vi "Robot Main.vi"() -> ()   [LabVIEW 2014]
doc: "This VI implements the framework and scheduler for your robotics program. It should not be necessary to modify the framework. You are expected to add your code to the VIs called from Robot Main - the ones located in the Team Code folder within the project."
uses:
  <vilib>/Rock Robotics/WPI/Camera/WPI_CameraImageSize.ctl
  TypeDefs/SRE Enum.ctl
  <vilib>/Rock Robotics/WPI/DriverStation/WPI_DriverStationDerivedRobotMode.ctl
  Support Code/Robot Global Data.vi
  <vilib>/Rock Robotics/Network Tables/SD Read Boolean.vi
panel:
  in  "Limit":dbl=0.45
  in  "Image Size":T1=enum."320x240"
  in  "Enable Vision":bool
  in  "Finish":bool
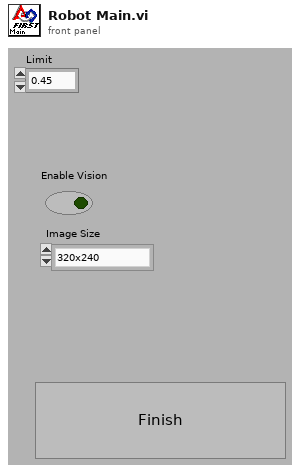
[diagram p1: front panel]
types:
  T1 = typedef "WPI_CameraImageSize.ctl" = enum16{"640x480", "320x240", "160x120", "Custom"}
  T2 = typedef "WPI_DriverStationDerivedRobotMode.ctl" = enum16{"Init", "Execute", "Stop"}
  T3 = typedef "SRE Enum.ctl" = enum16{"Start", "Run", "End"}
  T4 = cluster{"Speed":dbl, "Direction":dbl, "Rotation":dbl}
  T5 = enum16{"High", "Middle", "Low", "Really Low", "Stopped"}
  T6 = typedef "WPI_DriverStationMatch Info.ctl" = cluster{"Autonomous Elapsed Seconds":dbl, "TeleOp Elapsed Seconds":dbl, "Disabled Elapsed Seconds":dbl, "Visited Autonomous":bool, "Visited TeleOp":bool, "Visited Disabled":bool, "Autonomous Settings":cluster{"Autonomous Style":enum16{"Iterative", "Independent"}, "VI Refnum":refnum<vi>}}
  T7 = typedef "WPI_DriverStationRobotMode2.ctl" = enum16{"Autonomous Disabled", "Autonomous Enabled", "Teleop Disabled", "Teleop Enabled", "Disconnected", "Finish", "Test Disabled", "Test Enabled", "Emergency Stopped"}
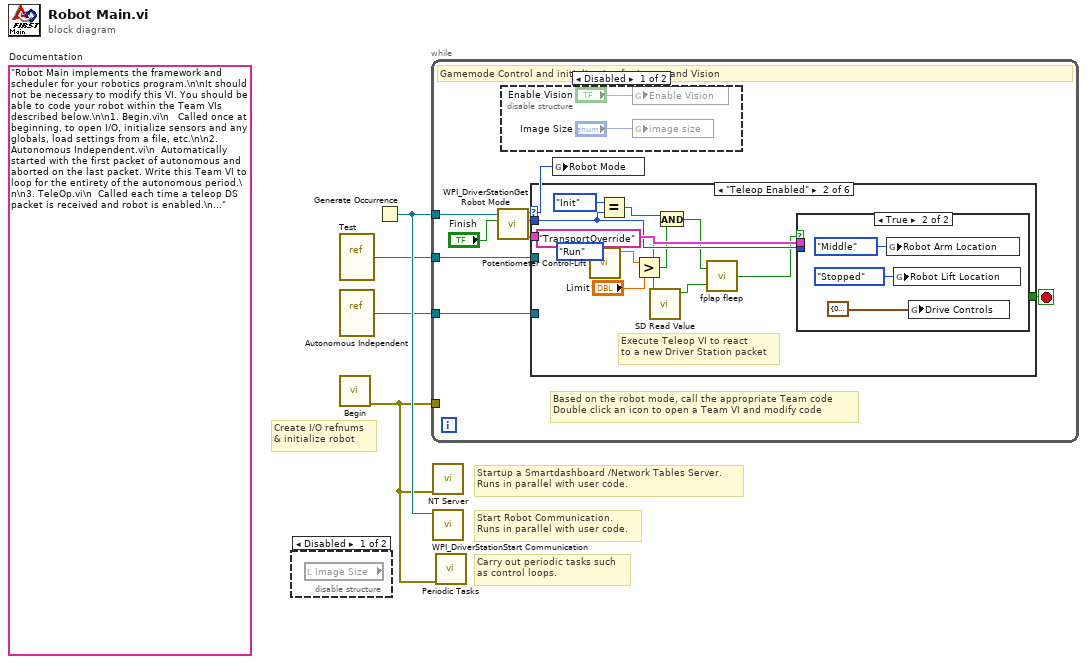
[diagram p0: block diagram]
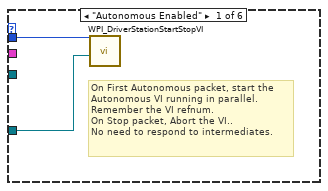
[diagram p4: hidden frame]
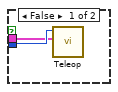
[diagram p5: hidden frame]
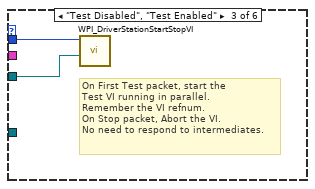
[diagram p6: hidden frame]
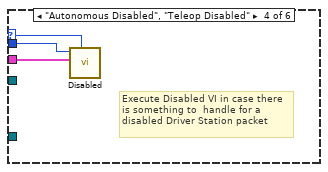
[diagram p7: hidden frame]
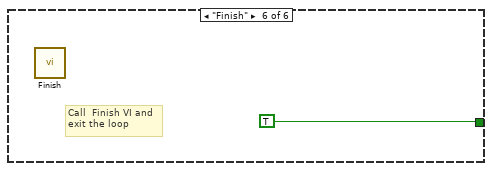
[diagram p9: hidden frame]
diagram:
  (unwired) "Robot Main implements the framework and scheduler for your robotics program.\n\nIt should not be necessary to modify this VI. You should be able to code your robot within the Team VIs described below.\n\n1. Begin.vi\n   Called once at beginning, to open I/O, initialize sensors and any globals, load settings from a file, etc.\n\n2. Autonomous Independent.vi\n  Automatically started with the first packet of autonomous and aborted on the last packet. Write this Team VI to loop for the entirety of the autonomous period.\n\n3. TeleOp.vi\n  Called each time a teleop DS packet is received and robot is enabled.\n\n4. Disabled.vi\n  Called each time a packet is received and the robot is disabled.\n\n5. Test.vi\n  Called Automatically started with the first test packet and aborted on the last. Modify this VI to carry out robot and sensor validation tests.\n\n6. Vision.vi\n  A parallel loop that acquires and processes camera images.\n\n7. PeriodicTasks.vi\n  Parallel loops running at user-defined rates.\n\n8. Finish.vi\n  Called before exiting, so you can save data, clean up I/O, etc.\n"  # Documentation
  # "Startup a Smartdashboard /Network Tables Server.\nRuns in parallel with user code."
  # "Carry out periodic tasks such\nas control loops."
  # "Create I/O refnums\n& initialize robot"
  # "Start Robot Communication.\nRuns in parallel with user code."
  n1 = disable-structure shown="Disabled" {
    frame Disabled {
      n2 = local read "Image Size"() -> ()  [unwired: 1 out]
    }
    frame Enabled {
    }
  }
  n3 = vi-ref "Test.vi"() -> (w2:refnum<vi>)
  n4 = vi-ref "Autonomous Independent.vi"() -> (w3:refnum<vi>)
  n5 = call "Begin.vi"() -> ("error in (no error)"=w1:errorcluster)  [unwired: 1 in, 10 out]
  n6 = Generate Occurrence() -> (w4:refnum<k4>)
  n7 = while "Scheduling loop" {
    tunnel: w4 -> [w11]
    tunnel: w1 -> [_]
    tunnel: w3 -> [w7]
    tunnel: w2 -> [w6]
    stop <- w8 stop-if-true
    # "Based on the robot mode, call the appropriate Team code\nDouble click an icon to open a Team VI and modify code"
    # "Gamemode Control and initialization for Image and Vision"
    n8 = call <vilib>:"WPI_DriverStationGet Robot Mode.vi"("Finish"="Finish", "DS Occurrence"=w11) -> ("Match Info out"=w9:T6, "Call Context"=w12:T2, "Robot Mode"=w5:T7)  [unwired: 7 out]
    n9 = disable-structure shown="Disabled" {
      frame Disabled {
        n10 = global write "Robot Global Data.vi" "Enable Vision"("Enable Vision") -> ()
        n11 = global write "Robot Global Data.vi" "image size"("Image Size") -> ()
      }
      frame Enabled {
      }
    }
    n12 = case shown="\"Teleop Enabled\"" w5 {
      selector: w5 -> [_ _ _ w36 _ _]
      tunnel: w12 -> [w16 w24 w35 w38 _ _]
      tunnel: w9 -> [_ w28 _ w37 _ _]
      tunnel: [_ _ _ _ _ TRUE] -> w8
      tunnel: w7 -> [w15 _ _ _ _ _]
      tunnel: w6 -> [_ _ w34 _ _ _]
      frame "Autonomous Enabled" {
        # "On First Autonomous packet, start the\nAutonomous VI running in parallel.\nRemember the VI refnum.\nOn Stop packet, Abort the VI..\nNo need to respond to intermediates."
        n13 = call <vilib>:"WPI_DriverStationStartStopVI.vi"("VI in"=w15, "Call Context"=w16) -> ()  [unwired: 10 in]
      }
      frame "Teleop Enabled" {
        # "Execute Teleop VI to react\nto a new Driver Station packet"
        n14 = call "Potentiometer Control-Lift.vi"("Enum"=SRE_Enum."Run") -> ("Normalized Value"=w26:dbl)  [unwired: 10 in]
        n15 = Equal?(x=WPI_DriverStationDerivedRobotMode."Init", y=w24) -> (x = y?=w22:bool)
        n16 = Greater?(x=w26, y="Limit") -> (0:w21:bool)
        n17 = call-poly <vilib>:"SD Read Value.vi"("Name"="TransportOverride") -> ("Boolean"=w17:bool)  [unwired: 8 in, 2 out]
        n18 = And(x=w22, y=w21) -> (x .and. y?=w20:bool)
        n19 = call "fplap fleep.vi"("False"=w17, "True"=w20) -> ("State"=w19:bool)
        n20 = case shown="True" w19 {
          tunnel: w24 -> [w30 _]
          tunnel: w28 -> [w29 _]
          frame False {
            n21 = call "Teleop.vi"("Match Info"=w29, "Call Context"=w30) -> ()  [unwired: 1 in, 9 out]
          }
          frame True {
            n22 = global write "Robot Global Data.vi" "Robot Arm Location"(enum16{"High", "Middle", "Low", "Noodle"}."Middle" ("Robot Arm Location")) -> ()
            n23 = global write "Robot Global Data.vi" "Robot Lift Location"(T5."Stopped" ("Robot Lift Location")) -> ()
            n24 = global write "Robot Global Data.vi" "Drive Controls"(T4 {"Speed"=0.0, "Direction"=0.0, "Rotation"=0.0} ("Drive Controls")) -> ()
          }
        }
      }
      frame "Test Disabled", "Test Enabled" {
        # "On First Test packet, start the\nTest VI running in parallel.\nRemember the VI refnum.\nOn Stop packet, Abort the VI.\nNo need to respond to intermediates."
        n25 = call <vilib>:"WPI_DriverStationStartStopVI.vi"("VI in"=w34, "Call Context"=w35) -> ()  [unwired: 10 in]
      }
      frame "Autonomous Disabled", "Teleop Disabled" {
        # "Execute Disabled VI in case there\nis something to  handle for a\ndisabled Driver Station packet"
        n26 = call "Disabled.vi"("Robot Mode"=w36, "Match Info"=w37, "Call Context"=w38) -> ()  [unwired: 1 in, 8 out]
      }
      frame "Disconnected", Default {
        # "Driver Station packet didn't arrive.\nPossibly useful for diagnostics"
      }
      frame "Finish" {
        # "Call  Finish VI and\nexit the loop"
        n27 = call "Finish.vi"() -> ()  [unwired: 1 in, 7 out]
      }
    }
    n28 = global write "Robot Global Data.vi" "Robot Mode"(w5) -> ()
  }
  n29 = call <vilib>:"NT Server.vi"("error in (no error)"=w1) -> ()  [unwired: 11 in]
  n30 = call <vilib>:"WPI_DriverStationStart Communication.vi"("occurrence"=w4) -> ()  [unwired: 1 in, 10 out]
  n31 = call "Periodic Tasks.vi"("error in"=w1) -> ()  [unwired: 1 in, 10 out]
